vi "Update Pixel Colour.vi"(4 "Colour":u32(colorbox), 8 "Column":i32, 10 "Current Row":i32, 11 "Pixel Data in in":u32[][](array[numeric])) -> (3 "Pixel Data out":u32[][](array[numeric]))   [LabVIEW 2022 SP3, in "Raster.lvlib"]
uses:
  Raster.lvlib
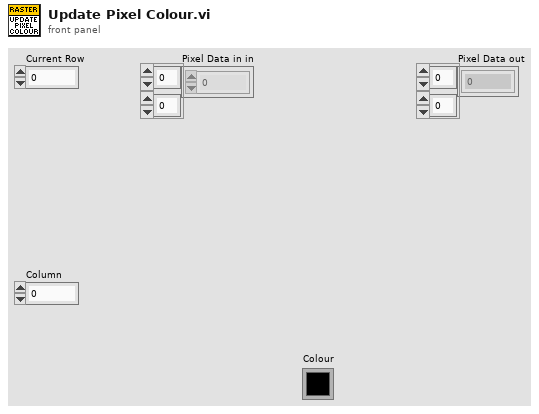
[diagram p1: front panel]
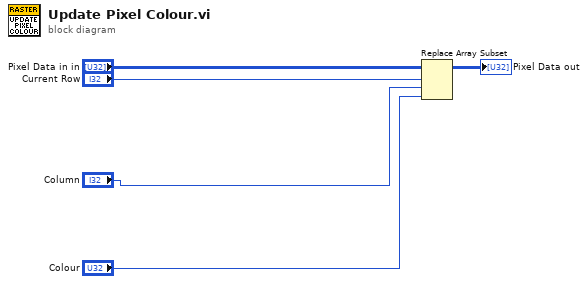
[diagram p0: block diagram]
diagram:
  n1 = Replace Array Subset(array="Pixel Data in in", new element="Colour", index (row)="Current Row", index (col)="Column") -> (→"Pixel Data out":u32[][])
